vi "CT-Create.vi"(0 "HCT Runtime in":T1, 7 "F0 (Hz)":dbl, 9 "Fs (Hz)":dbl, 11 "error in (no error)":errorcluster) -> (4 "HCT Runtime out":T1, 8 "HCT":dbl[](array[numeric]), 15 "error out":errorcluster)   [LabVIEW 2015]
uses:
  Utility VIs/Math VIs/LinSpace (x0-dx-npts).vi
  HCT-Runtime Data.ctl
panel:
  in  "Npts":i32
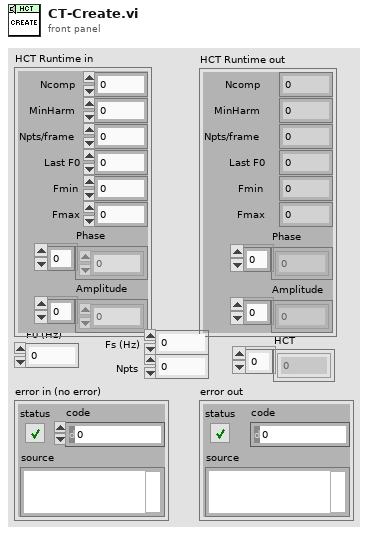
[diagram p1: front panel]
types:
  T1 = typedef "HCT-Runtime Data.ctl" = cluster{"Ncomp":i32, "MinHarm":i32, "Phase":dbl[], "Amplitude":dbl[], "Npts/frame":i32, "Last F0":dbl, "Fmin":dbl, "Fmax":dbl}
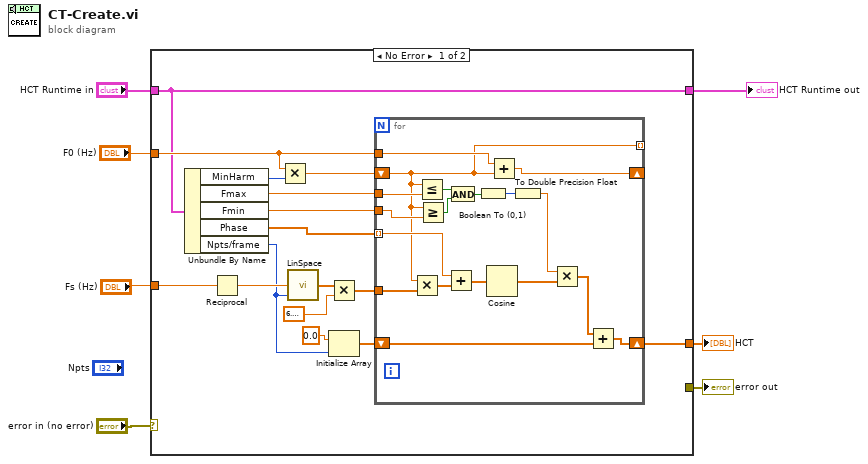
[diagram p0: block diagram]
diagram:
  n1 = case shown="No Error" "error in (no error)" {
    selector: "error in (no error)" -> [_ w42]
    tunnel: "HCT Runtime in" -> [w20 _]
    tunnel: [w20 _] -> w4
    tunnel: "F0 (Hz)" -> [w21 _]
    tunnel: [_ w42] -> w7
    tunnel: "Fs (Hz)" -> [w18 _]
    tunnel: [w10 _] -> w1
    frame No Error {
      n2 = Unbundle By Name(w20) -> ("MinHarm"=w23:i32, "Fmax"=w9:dbl, "Fmin"=w8:dbl, "Phase"=w11:dbl[], "Npts/frame"=w12:i32)
      n3 = Reciprocal(x=w18) -> (1/x=w19:dbl)
      n4 = Multiply(x=w21, y=w23) -> (x*y=w22:dbl)
      n5 = call-poly "LinSpace.vi"("npts"=w12, "dx"=w19) -> ("Array"=w17:dbl[])  [unwired: 2 in, 1 out]
      n6 = Multiply(x=w17, y=6.283185307179586) -> (x*y=w15:dbl[])
      n7 = Initialize Array(0.0 ("element"), w12) -> (w13:dbl[])
      n8 = for {
        shift-right: [w41] -> _
        shift-left: w22 -> [w24]
        tunnel: w21 -> [w40]
        tunnel: w15 -> [w39]
        shift-right: [w33] -> w10
        shift-left: w13 -> [w34]
        tunnel: w11 -> [w38] mode=indexing
        tunnel: w9 -> [w29]
        tunnel: w8 -> [w28]
        tunnel: [w24] -> _ mode=indexing
        n9 = Multiply(x=w24, y=w39) -> (x*y=w37:dbl[])
        n10 = Less Or Equal?(x=w24, y=w29) -> (x <= y?=w27:bool)
        n11 = Greater Or Equal?(x=w24, y=w28) -> (x >= y?=w26:bool)
        n12 = Add(x=w38, y=w37) -> (x+y=w36:dbl[])
        n13 = And(x=w27, y=w26) -> (x .and. y?=w25:bool)
        n14 = Boolean To (0,1)(Boolean=w25) -> (0, 1=w32:i16)
        n15 = Cosine(x=w36) -> (cos(x)=w35:dbl[])
        n16 = Add(x=w40, y=w24) -> (x+y=w41:dbl)
        n17 = To Double Precision Float(number=w32) -> (double precision float=w30:dbl)
        n18 = Multiply(x=w30, y=w35) -> (x*y=w31:dbl[])
        n19 = Add(x=w31, y=w34) -> (x+y=w33:dbl[])
      }
    }
    frame Error {
    }
  }
  "error out" <- w7
  "HCT Runtime out" <- w4
  "HCT" <- w1
